vi "Com Read serial with wait.vi"(4 "Ignore Visa Read Error\n-1073807298":bool, 6 "Clear Buffer initally(f)":bool, 7 "Stop String array":string[](array[string]), 8 "Error":errorcluster, 9 "Read Times":T1, 11 "Com":refnum<visa-resource-name>) -> (0 "Error Out":errorcluster, 1 "Status Out":T2, 2 "Read String Out":string, 3 "Com Out":refnum<visa-resource-name>)   [LabVIEW 2015]
uses:
  TypeDefs_Utility/ENUM_Com_Read Status.ctl
  TypeDefs_Utility/Cluster_Com_Read Times.ctl
panel:
  out "Bytes at Serial Port":u32
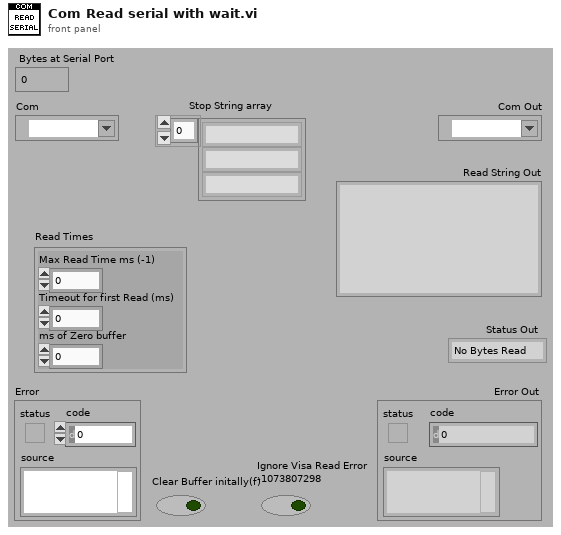
[diagram p1: front panel]
types:
  T1 = typedef "Cluster_Com_Read Times.ctl" = cluster{"Max Read Time ms (-1)":i32, "Timeout for first Read (ms)":u32, "ms of Zero buffer":u32}
  T2 = typedef "ENUM_Com_Read Status.ctl" = enum16{"No Bytes Read", "Bytes Read", "Stop String Read"}
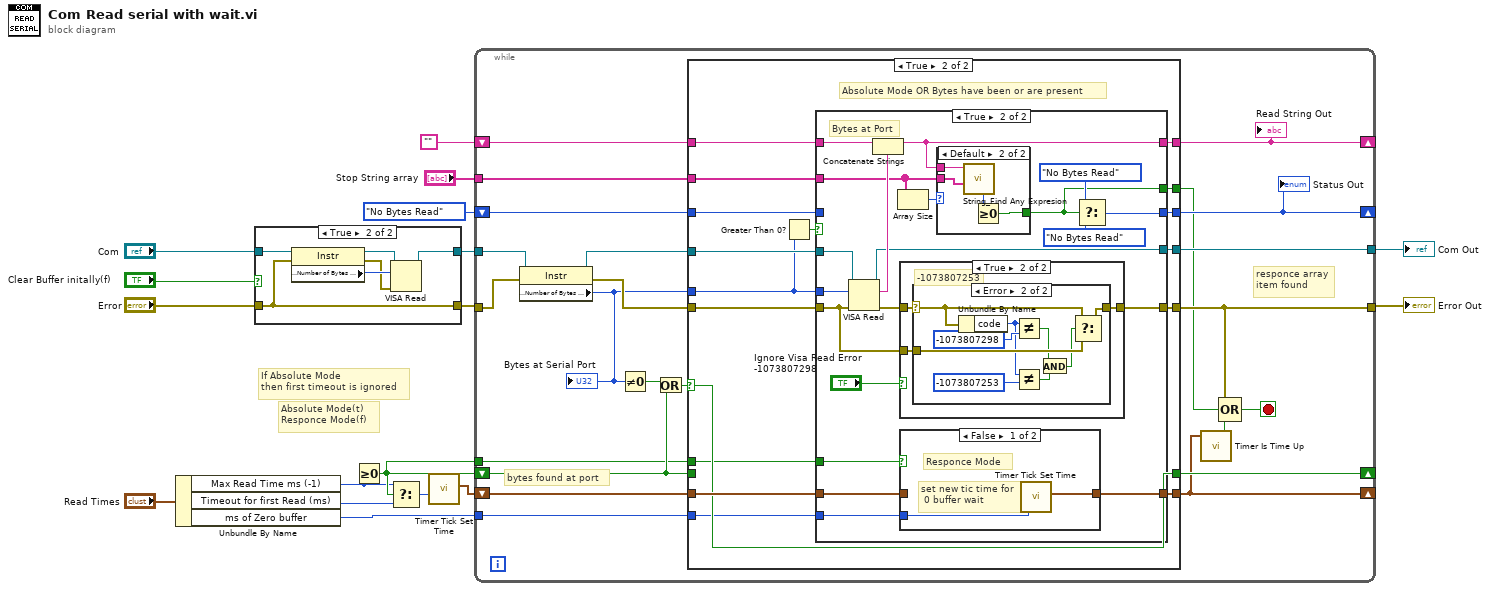
[diagram p0: block diagram]
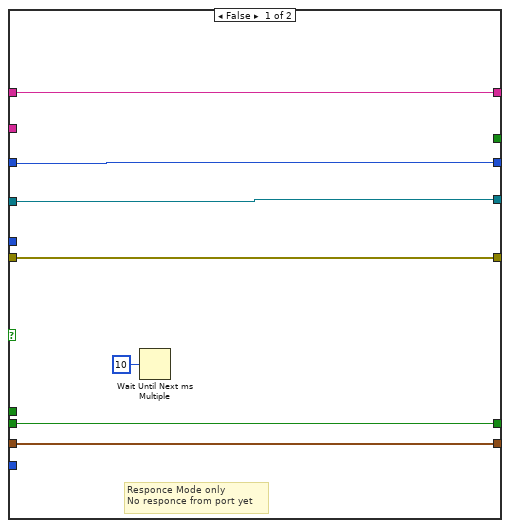
[diagram p3: hidden frame]
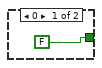
[diagram p7: hidden frame]
diagram:
  # "Absolute Mode(t)\nResponce Mode(f)"
  # "If Absolute Mode\nthen first timeout is ignored"
  n1 = Unbundle By Name("Read Times") -> ("Max Read Time ms (-1)"=w5:i32, "Timeout for first Read (ms)"=w4:u32, "ms of Zero buffer"=w7:u32)
  n2 = case shown="True" "Clear Buffer initally(f)" {
    tunnel: "Com" -> [w19 w25]
    tunnel: [w19 w22] -> w12
    tunnel: [w18 w20] -> w11
    tunnel: "Error" -> [w18 w20]
    frame False {
    }
    frame True {
      n3 = property class="Instr"(reference=w25, error in=w20) -> (reference out=w23:refnum<visa-resource-name>, error out=w21:errorcluster, "Serial Settings:Number of Bytes at Serial Port"=w24:u32)
      n4 = VISA Read(VISA resource name=w23, byte count=w24, error in (no error)=w21) -> (VISA resource name out=w22:refnum<visa-resource-name>)  [unwired: 3 out]
    }
  }
  n5 = Greater Or Equal To 0?(x=w5) -> (x >= 0?=w6:bool)
  n6 = Select(t=w5, s=w6, f=w4) -> (s? t:f=w3:u32)
  n7 = call "Timer Tick Set Time.vi"("Seconds till stop (ms)"=w3) -> ("Finish Time"=w2:timestamp)  [unwired: 5 in, 1 out]
  n8 = while {
    shift-left: "" -> [w38]
    shift-right: [w33] -> _
    shift-left: w6 -> [w39]
    shift-right: [w40] -> _
    shift-left: w2 -> [w43]
    shift-right: [w28] -> _
    tunnel: w11 -> [w47]
    tunnel: w12 -> [w48]
    tunnel: [w44] -> w16
    tunnel: [w30] -> w15
    tunnel: w7 -> [w36]
    shift-right: [w31] -> _
    shift-left: ENUM_Com_Read_Status."No Bytes Read" ("Status") -> [w35]
    tunnel: w6 -> [w34]
    tunnel: "Stop String array" -> [w32]
    stop <- w26 stop-if-true
    # "responce array\nitem found"
    # "bytes found at port"
    n9 = property class="Instr"(reference=w48, error in=w47) -> (reference out=w45:refnum<visa-resource-name>, error out=w46:errorcluster, "Serial Settings:Number of Bytes at Serial Port"=w37:u32)
    "Bytes at Serial Port" <- w37
    n10 = Not Equal To 0?(x=w37) -> (x != 0?=w41:bool)
    n11 = Or(x=w41, y=w39) -> (x .or. y?=w42:bool)
    n12 = case shown="True" w42 {
      selector: w42 -> [_ w70]
      tunnel: w46 -> [w54 w67]
      tunnel: [w54 w66] -> w30
      tunnel: w45 -> [w55 w68]
      tunnel: [w55 w65] -> w44
      tunnel: w37 -> [_ w62]
      tunnel: w43 -> [w49 w72]
      tunnel: [w49 w71] -> w28
      tunnel: [w53 w70] -> w40
      tunnel: w39 -> [w53 _]
      tunnel: w38 -> [w52 w64]
      tunnel: [w52 w63] -> w33
      tunnel: w36 -> [_ w61]
      tunnel: [w51 w60] -> w31
      tunnel: w35 -> [w51 w57]
      tunnel: w34 -> [_ w59]
      tunnel: w32 -> [_ w58]
      tunnel: [_ w56] -> w29
      frame False {
        # "Responce Mode only\nNo responce from port yet"
        n13 = Wait Until Next ms Multiple(millisecond multiple=u32 10) -> ()  [unwired: 1 out]
      }
      frame True {
        # "Absolute Mode OR Bytes have been or are present"
        n14 = Greater Than 0?(x=w62) -> (x > 0?=w69:bool)
        n15 = case shown="True" w69 {
          tunnel: [w73 w82] -> w71
          tunnel: w72 -> [w73 w90]
          tunnel: w62 -> [_ w97]
          tunnel: w68 -> [w77 w96]
          tunnel: w67 -> [w76 w86]
          tunnel: [w76 w87] -> w66
          tunnel: [w77 w85] -> w65
          tunnel: w64 -> [w75 w95]
          tunnel: [w75 w92] -> w63
          tunnel: w61 -> [_ w94]
          tunnel: [w74 w79] -> w60
          tunnel: w57 -> [w74 _]
          tunnel: w59 -> [_ w91]
          tunnel: w58 -> [_ w83]
          tunnel: [_ w78] -> w56
          frame False {
            # "NO Bytes at Port"
          }
          frame True {
            # "Bytes at Port"
            n16 = VISA Read(VISA resource name=w96, byte count=w97, error in (no error)=w86) -> (VISA resource name out=w85:refnum<visa-resource-name>, read buffer=w93:string, error out=w88:errorcluster)  [unwired: 1 out]
            n17 = Concatenate Strings(w95, w93) -> (w92:string)
            n18 = Array Size(array=w83) -> (size(s)=w89:i32)
            n19 = case shown="True" "Ignore Visa Read Error\n-1073807298" {
              tunnel: w88 -> [w98 w101]
              tunnel: [w98 w100] -> w87
              tunnel: w86 -> [_ w99]
              frame False {
              }
              frame True {
                # "-1073807253"
                n20 = case shown="Error" w101 {
                  selector: w101 -> [w102 w110]
                  tunnel: [w102 w109] -> w100
                  tunnel: w99 -> [_ w111]
                  frame No Error {
                  }
                  frame Error {
                    n21 = Unbundle By Name(w110) -> ("code"=w107:i32)
                    n22 = Not Equal?(x=w107, y=-1073807298) -> (x != y?=w104:bool)
                    n23 = Not Equal?(x=w107, y=-1073807253) -> (x != y?=w105:bool)
                    n24 = And(x=w104, y=w105) -> (x .and. y?=w103:bool)
                    n25 = Select(t=w110, s=w103, f=w111) -> (s? t:f=w109:errorcluster)
                  }
                }
              }
            }
            n26 = case shown="False" w91 {
              tunnel: w94 -> [w118 _]
              tunnel: [w117 w119] -> w82
              tunnel: w90 -> [_ w119]
              frame False {
                # "Responce Mode"
                # "set new tic time for\n 0 buffer wait"
                n27 = call "Timer Tick Set Time.vi"("Seconds till stop (ms)"=w118) -> ("Finish Time"=w117:timestamp)  [unwired: 5 in, 1 out]
              }
              frame True {
                # "Absolute Mode"
              }
            }
            n28 = case shown="Default" w89 {
              tunnel: w92 -> [_ w116]
              tunnel: w83 -> [_ w115]
              tunnel: [FALSE w113] -> w78
              frame 0 {
              }
              frame Default {
                n29 = call "String_Find Any Expresion.vi"("Match Strings"=w115, "String"=w116) -> ("Offset Past Match Out"=w114:i32)  [unwired: 5 in, 4 out]
                n30 = Greater Or Equal To 0?(x=w114) -> (x >= 0?=w113:bool)
              }
            }
            n31 = Select(t=ENUM_Com_Read_Status."No Bytes Read" ("Status"), s=w78, f=ENUM_Com_Read_Status."No Bytes Read" ("Status")) -> (s? t:f=w79:T2)
          }
        }
      }
    }
    "Read String Out" <- w33
    "Status Out" <- w31
    n32 = call "Timer Is Time Up.vi"("Finish Time"=w28) -> ("Time Complete"=w27:bool)  [unwired: 2 in, 2 out]
    n33 = Compound Arithmetic op=OR(w30, w29, w27) -> (w26:bool)
  }
  "Com Out" <- w16
  "Error Out" <- w15
